vi "main.vi"() -> ()   [LabVIEW 2016]
uses:
  <userlib>/ROS for LabVIEW Software/ROS/Code/SubVIs/_ROSDirection.ctl
  <userlib>/ROS for LabVIEW Software/ROS/Code/Console/Servers/ServerSubs/TopicDef.ctl
  <vilib>/myRIO/Express VI/Onboard Devices/LED/LED Express VI.xnode
  <vilib>/myRIO/Instrument Drivers/Onboard IO/DIO/vis/Write.vi
  <vilib>/myRIO/Instrument Drivers/Onboard IO/DIO/DIO.lvlib
  <vilib>/myRIO/Common/Instrument Driver Framework/myRIO v1.0/DIO/typedefs/DIO Channels Enum.ctl
  <vilib>/myRIO/Common/Instrument Driver Framework/myRIO v1.0/DIO/typedefs/DIO Channels List.ctl
  <vilib>/myRIO/Common/Instrument Driver Framework/Utilities/typedefs/Generic FPGA Reference.ctl
  <vilib>/myRIO/Common/Instrument Driver Framework/Utilities/typedefs/myRIO v1.0 Reference.ctl
  <vilib>/myRIO/Common/Instrument Driver Framework/Utilities/typedefs/Hardware Version Enum.ctl
  <vilib>/myRIO/Common/Instrument Driver Framework/Utilities/typedefs/myRIO Generic Hardware Reference.ctl
  <vilib>/myRIO/Instrument Drivers/Onboard IO/DIO/typedefs/DIO Reference.ctl
  <vilib>/myRIO/Instrument Drivers/Onboard IO/DIO/vis/myRIO DIO Open.xnode
  <vilib>/myRIO/Common/Instrument Driver Framework/Utilities/vis/Is FPGA Ref Available.vi
  <vilib>/myRIO/Common/Instrument Driver Framework/roboRIO v1.0/DIO/vis/roboRIO v1.0 Open DIO.vi
  <vilib>/userdefined/High Color/nirio_resource_hc.ctl
  <vilib>/myRIO/Express VI/Onboard IO/PWM/PWM Express VI.xnode
  <vilib>/myRIO/Instrument Drivers/Onboard IO/PWM/vis/Set Duty Cycle and Frequency.vi
  <vilib>/myRIO/Instrument Drivers/Onboard IO/PWM/PWM.lvlib
  <vilib>/myRIO/Instrument Drivers/Onboard IO/PWM/typedefs/PWM Configuration.ctl
  <vilib>/myRIO/Common/Instrument Driver Framework/myRIO v1.0/PWM/typedefs/PWM Channels Enum.ctl
  <vilib>/myRIO/Instrument Drivers/Onboard IO/PWM/typedefs/PWM Reference.ctl
  <vilib>/myRIO/Instrument Drivers/Onboard IO/PWM/vis/myRIO PWM Open.xnode
  <vilib>/myRIO/Common/Instrument Driver Framework/roboRIO v1.0/PWM/vis/roboRIO v1.0 Open PWM.vi
  <userlib>/ROS for LabVIEW Software/ROS/MessageParsing/std_msgs/subs/parse_u8_scalar.vi
panel:
  out "set_steering":dbl
  out "set_speed":dbl
  out "error out":errorcluster
  out "Stopped?":bool
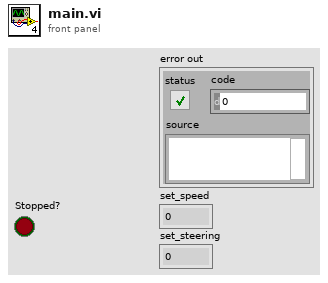
[diagram p1: front panel]
types:
  T1 = typedef "PWM.lvlib/PWM Reference.ctl" = cluster{"myRIO Reference":T2, "PWM Channels Enum":T6, "PWM Configuration":T7}
  T2 = typedef "myRIO Generic Hardware Reference.ctl" = cluster{"myRIO Model":T3, "myRIO Hardware Reference":T4}
  T3 = typedef "Hardware Version Enum.ctl" = enum16{"Unknown", "myRIO-1900", "myRIO-1950", "roboRIO", "NI ELVIS RIO CM"}
  T4 = typedef "myRIO v1.0 Reference.ctl" = cluster{"Generic FPGA Reference":T5, "Allow multiple opens":bool}
  T5 = typedef "Generic FPGA Reference.ctl" = refnum<k20>
  T6 = typedef "PWM Channels Enum.ctl" = enum16{"Not Connected", "C/PWM0", "C/PWM1", "A/PWM0", "A/PWM1", "A/PWM2", "B/PWM0", "B/PWM1", "B/PWM2", "PWM/PWM0", "PWM/PWM1", "PWM/PWM2", "PWM/PWM3", "PWM/PWM4", "PWM/PWM5", "PWM/PWM6", "PWM/PWM7", "PWM/PWM8", "PWM/PWM9"}
  T7 = typedef "PWM.lvlib/PWM Configuration.ctl" = cluster{"Frequency":dbl, "Duty Cycle":dbl}
  T8 = typedef "nirio_resource_hc.ctl" = tag
  T9 = typedef "TopicDef.ctl" = cluster{"Topic":string, "Type":string, "Action":T10, "Update (ms)":u16, "queue size":u16}
  T10 = typedef "_ROSDirection.ctl" = enum16{"Node", "Publisher", "Subscriber", "ServiceClient", "ServiceProvider"}
  T11 = typedef "DIO.lvlib/DIO Reference.ctl" = cluster{"myRIO Reference":T2, "DIO Channels List":T12}
  T12 = typedef "DIO Channels List.ctl" = T13[]
  T13 = typedef "DIO Channels Enum.ctl" = enum16{"Not Connected", "C/DIO0", "C/DIO1", "C/DIO2", "C/DIO3", "C/DIO4", "C/DIO5", "C/DIO6", "C/DIO7", "A/DIO0", "A/DIO1", "A/DIO2", "A/DIO3", "A/DIO4", "A/DIO5", "A/DIO6", "A/DIO7", "A/DIO8", "A/DIO9", "A/DIO10", "A/DIO11", "A/DIO12", "A/DIO13", "A/DIO14", "A/DIO15", "B/DIO0", "B/DIO1", "B/DIO2", "B/DIO3", "B/DIO4", "B/DIO5", "B/DIO6", "B/DIO7", "B/DIO8", "B/DIO9", "B/DIO10", "B/DIO11", "B/DIO12", "B/DIO13", "B/DIO14", "B/DIO15", "LED0", "LED1", "LED2", "LED3", "Button0", "DIO/DIO0", "DIO/DIO1", "DIO/DIO2", "DIO/DIO3", "DIO/DIO4", "DIO/DIO5", "DIO/DIO6", "DIO/DIO7", "DIO/DIO8", "DIO/DIO9", "SPI/CS0", "SPI/CS1", "SPI/CS2", "SPI/CS3", "LED RADIO (Green)", "LED RADIO (Red)", "LED COMM (Green)", "LED COMM (Red)", "LED MODE (Green)", "LED MODE (Red)"}
  T14 = typedef "_ROSControl.ctl" = cluster{"topic port":u16, "Node":string, "topic":string, "type":string, "node port":u16, "error ":errorcluster, "Direction":T10, "Update (ms)":u16, "FIFO size":u16}
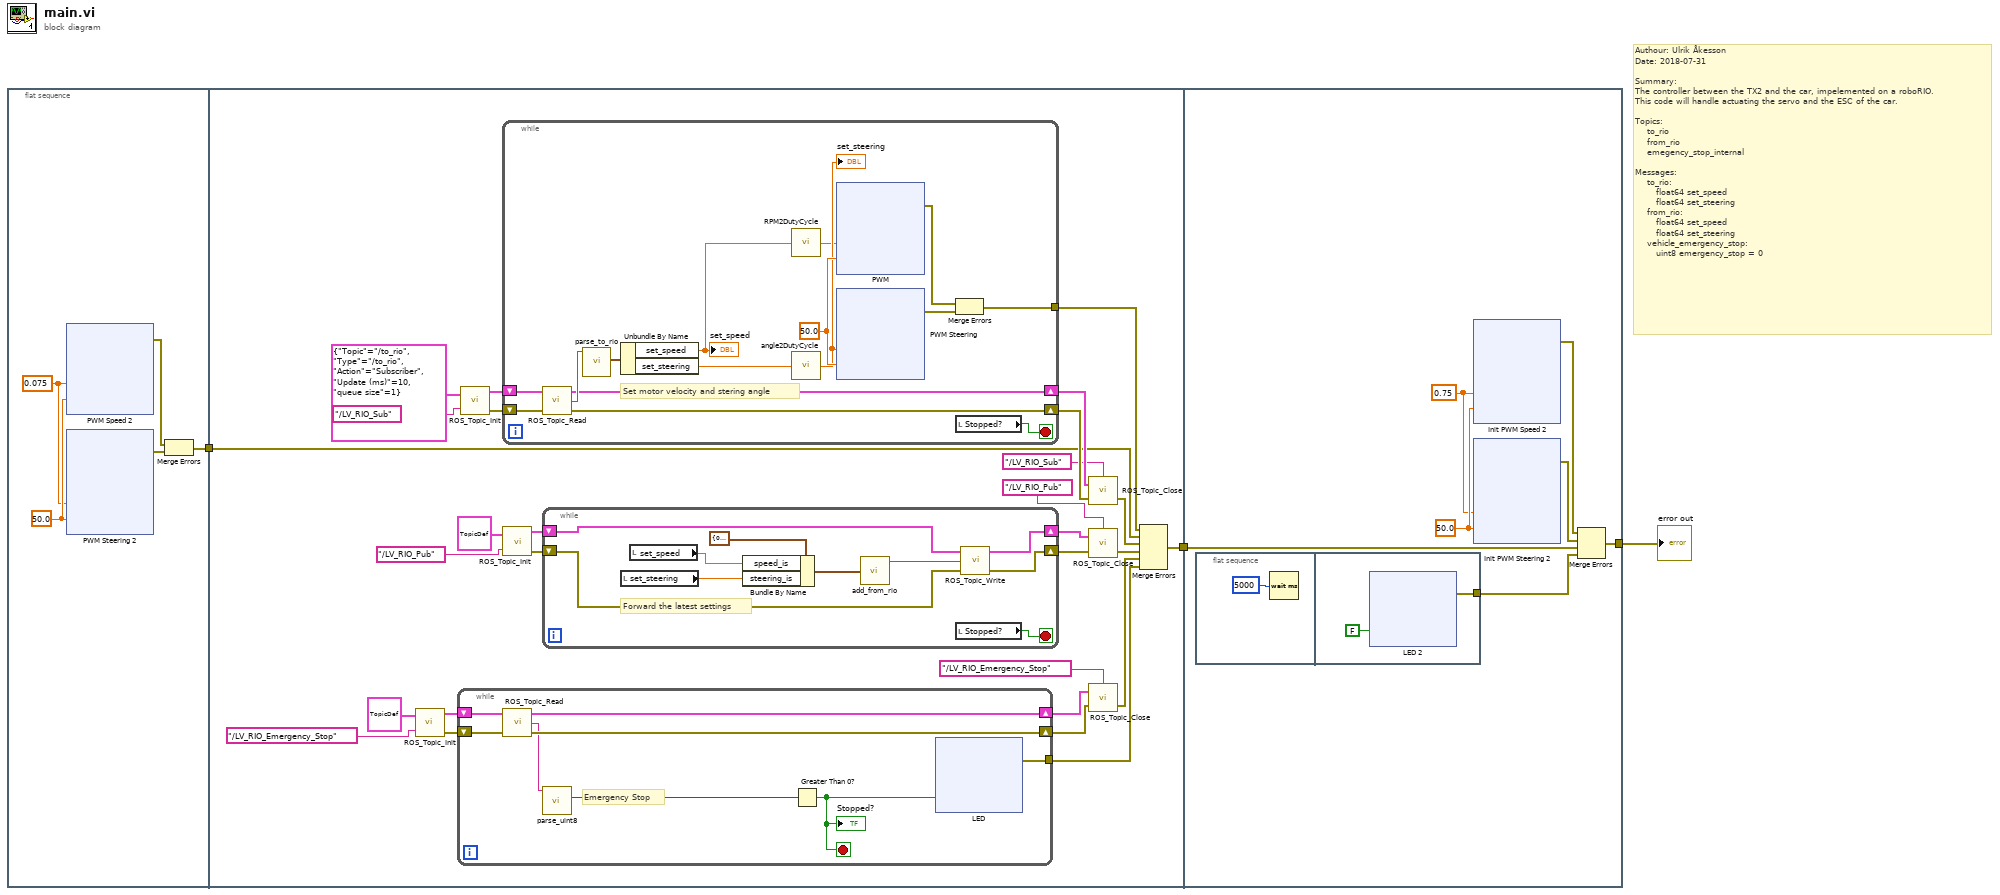
[diagram p0: block diagram]
diagram:
  # "Authour: Ulrik Åkesson\nDate: 2018-07-31\n\nSummary:\nThe controller between the TX2 and the car, impelemented on a roboRIO.\nThis code will handle actuating the servo and the ESC of the car.\n\nTopics:\n    to_rio\n    from_rio\n    emegency_stop_internal\n\nMessages:\n    to_rio:\n       float64 set_speed\n       float64 set_steering\n    from_rio:\n       float64 set_speed\n       float64 set_steering\n    vehicle_emergency_stop:\n       uint8 emergency_stop = 0"
  n1 = flat-sequence {
    tunnel: [w4] -> w3
    tunnel: w3 -> [w81]
    tunnel: [w80] -> w2
    tunnel: w2 -> [w247]
    tunnel: [w246] -> w1
    frame #0 {
      w7 = 0.075
      w8 = 50.0
      n2 = xnode "PWM Speed 2"("Duty Cycle"=w7, "Frequency [Hz]"=w8) -> ("error out"=w6:errorcluster)  [unwired: 1 in]
      n3 = xnode "PWM Steering 2"("Duty Cycle"=w7, "Frequency [Hz]"=w8) -> ("error out"=w5:errorcluster)  [unwired: 1 in]
      n4 = Merge Errors(w6, w5) -> (w4:errorcluster)
    }
    frame #1 {
      n5 = call <userlib>:"ROS_Topic_Init.vi"("Definitions"=T9 {"Topic"="/emergency_stop_internal", "Type"="/vehicle_emergency_stop", "Action"=enum."Subscriber", "Update (ms)"=100, "queue size"=1}, "node"="/LV_RIO_Emergency_Stop") -> ("ROS out"=w98:T14, "error out"=w97:errorcluster)  [unwired: 1 in]
      n6 = while {
        shift-right: [w112] -> w96
        shift-left: w98 -> [w114]
        shift-right: [w111] -> w95
        shift-left: w97 -> [w113]
        tunnel: [w107] -> w82
        stop <- w108 stop-if-true
        # "Emergency Stop"
        n7 = call <userlib>:"ROS_Topic_Read.vi"("error in (no error)"=w113, "ROS in"=w114) -> ("error out"=w111:errorcluster, "Reply"=w110:string, "ROS out"=w112:T14)  [unwired: 1 in]
        n8 = call-poly <userlib>:"parse_uint8.vi"("msg in"=w110) -> ("number"=w109:u8)  [unwired: 4 in, 2 out]
        n9 = Greater Than 0?(x=w109) -> (x > 0?=w108:bool)
        "Stopped?" <- w108
        n10 = xnode "LED"("MODE (Red)"=w108) -> ("error out"=w107:errorcluster)  [unwired: 1 in]
      }
      n11 = call <userlib>:"ROS_Topic_Init.vi"("Definitions"=T9 {"Topic"="/to_rio", "Type"="/to_rio", "Action"=enum."Subscriber", "Update (ms)"=10, "queue size"=1}, "node"="/LV_RIO_Sub") -> ("ROS out"=w106:T14, "error out"=w105:errorcluster)  [unwired: 1 in]
      n12 = while {
        shift-right: [w171] -> w104
        shift-left: w106 -> [w173]
        shift-right: [w170] -> w103
        shift-left: w105 -> [w172]
        tunnel: [w164] -> w79
        stop <- w169 stop-if-true
        w167 = 50.0 ("Frequency [Hz]")
        # "Set motor velocity and stering angle"
        n13 = call <userlib>:"ROS_Topic_Read.vi"("error in (no error)"=w172, "ROS in"=w173) -> ("error out"=w170:errorcluster, "Reply"=w174:string, "ROS out"=w171:T14)  [unwired: 1 in]
        n14 = call "parse_to_rio.vi"("msg in"=w174) -> ("to_rio"=w168:cluster{"set_speed":dbl, "set_steering":dbl})  [unwired: 4 in, 2 out]
        n15 = Unbundle By Name(w168) -> ("set_speed"=w160:dbl, "set_steering"=w163:dbl)
        "set_speed" <- w160
        n16 = call "RPM2DutyCycle.vi"("Speed"=w160) -> ("Duty Cycle"=w161:dbl)
        n17 = call "angle2DutyCycle.vi"("Steering Angle"=w163) -> ("Duty Cycle"=w162:dbl)
        "set_steering" <- w162
        n18 = xnode "PWM"("Duty Cycle"=w161, "Frequency [Hz]"=w167) -> ("error out"=w166:errorcluster)  [unwired: 1 in]
        n19 = xnode "PWM Steering"("Duty Cycle"=w162, "Frequency [Hz]"=w167) -> ("error out"=w165:errorcluster)  [unwired: 1 in]
        n20 = Merge Errors(w166, w165) -> (w164:errorcluster)
        n21 = local read "Stopped?"() -> (w169:bool)
      }
      n22 = call <userlib>:"ROS_Topic_Init.vi"("Definitions"=T9 {"Topic"="/from_rio", "Type"="/from_rio", "Action"=enum."Publisher", "Update (ms)"=10, "queue size"=1}, "node"="/LV_RIO_Pub") -> ("ROS out"=w100:T14, "error out"=w99:errorcluster)  [unwired: 1 in]
      n23 = while {
        shift-right: [w158] -> w102
        shift-left: w100 -> [w156]
        shift-right: [w157] -> w101
        shift-left: w99 -> [w155]
        stop <- w154 stop-if-true
        # "Forward the latest settings"
        n24 = local read "set_steering"() -> (w151:dbl)
        n25 = local read "set_speed"() -> (w152:dbl)
        n26 = Bundle By Name(cluster=cluster{"speed_is":dbl, "steering_is":dbl} {"speed_is"=0.0, "steering_is"=0.0} ("from_rio"), "speed_is"=w152, "steering_is"=w151) -> (w150:cluster{"speed_is":dbl, "steering_is":dbl})
        n27 = call "add_from_rio.vi"("from_rio"=w150) -> ("msg out"=w159:string)  [unwired: 4 in]
        n28 = local read "Stopped?"() -> (w154:bool)
        n29 = call <userlib>:"ROS_Topic_Write.vi"("error in (no error)"=w155, "Msg in"=w159, "ROS in"=w156) -> ("error out"=w157:errorcluster, "ROS out"=w158:T14)  [unwired: 1 in]
      }
      n30 = call <userlib>:"ROS_Topic_Close.vi"("error in"=w103, "ROS in"=w104, "node"="/LV_RIO_Sub") -> ("error out"=w94:errorcluster)  [unwired: 1 in]
      n31 = call <userlib>:"ROS_Topic_Close.vi"("error in"=w101, "ROS in"=w102, "node"="/LV_RIO_Pub") -> ("error out"=w93:errorcluster)  [unwired: 1 in]
      n32 = call <userlib>:"ROS_Topic_Close.vi"("error in"=w95, "ROS in"=w96, "node"="/LV_RIO_Emergency_Stop") -> ("error out"=w92:errorcluster)  [unwired: 1 in]
      n33 = Merge Errors(w79, w81, w94, w93, w92, w82) -> (w80:errorcluster)
    }
    frame #2 {
      w250 = 0.75
      w251 = 50.0
      n34 = flat-sequence {
        tunnel: [w253] -> w245
        frame #0 {
          n35 = Wait (ms)(milliseconds to wait=u32 5000) -> ()  [unwired: 1 out]
        }
        frame #1 {
          n36 = xnode "LED 2"("MODE (Red)"=FALSE) -> ("error out"=w253:errorcluster)  [unwired: 1 in]
        }
      }
      n37 = xnode "Init PWM Speed 2"("Duty Cycle"=w250, "Frequency [Hz]"=w251) -> ("error out"=w249:errorcluster)  [unwired: 1 in]
      n38 = xnode "Init PWM Steering 2"("Duty Cycle"=w250, "Frequency [Hz]"=w251) -> ("error out"=w248:errorcluster)  [unwired: 1 in]
      n39 = Merge Errors(w249, w248, w247, w245) -> (w246:errorcluster)
    }
  }
  "error out" <- w1
